vi "fgv_USBSrial-w.vi"() -> ()   [LabVIEW 2019]
panel:
  out "concatenated string":string
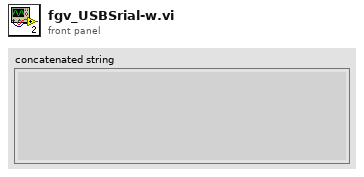
[diagram p1: front panel]
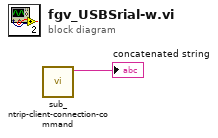
[diagram p0: block diagram]
diagram:
  n1 = call "sub_ntrip-client-connection-command.vi"() -> ("hex"=→"concatenated string":string)  [unwired: 11 in]
